vi "Get Module Execution Status.vi"(8 "error in":errorcluster) -> (0 "error out":errorcluster)   [LabVIEW 2025, in "Number Pad.lvlib"]
doc: "Fire the Get Module Execution Status request.\n_____\nBased on DQMH Dev Tools: Project Template 7.1.0.1503."
uses:
  Number Pad.lvlib
  Get Module Execution Status Argument--cluster.ctl
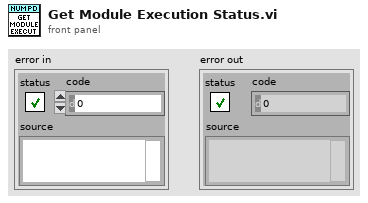
[diagram p1: front panel]
types:
  T1 = typedef "Number Pad.lvlib/Get Module Execution Status Argument--cluster.ctl" = cluster{"Running?":bool}
  T2 = typedef "Number Pad.lvlib/Request Events--cluster.ctl" = cluster{"Stop Module":refnum<user-event>, "Show Panel":refnum<user-event>, "Hide Panel":refnum<user-event>, "Get Module Execution Status":refnum<user-event>, "Show Diagram":refnum<user-event>}
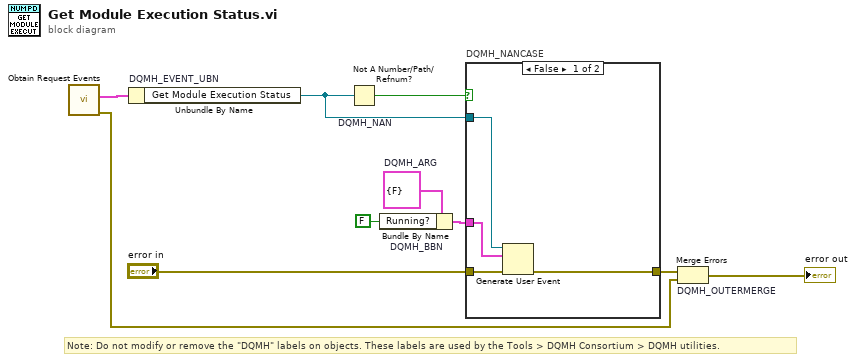
[diagram p0: block diagram]
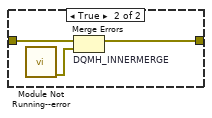
[diagram p2: hidden frame]
diagram:
  w4 = T1 {"Running?"=FALSE}  # DQMH_ARG
  # "Note: Do not modify or remove the \"DQMH\" labels on objects. These labels are used by the Tools > DQMH Consortium > DQMH utilities."
  n1 = call "Obtain Request Events.vi"() -> ("error out"=w2:errorcluster, "Number Pad Request Events"=w1:T2)  [unwired: 10 in]
  n2 = Unbundle By Name "DQMH_EVENT_UBN"(w1) -> ("Get Module Execution Status"=w5:refnum<user-event>)
  n3 = Not A Number/Path/Refnum? "DQMH_NAN"(number/path/refnum=w5) -> (NaN/Path/Refnum?=w6:bool)
  n4 = Bundle By Name "DQMH_BBN"(cluster=w4, "Running?"=FALSE) -> (w7:T1)
  n5 = case "DQMH_NANCASE" shown="False" w6 {
    tunnel: "error in" -> [w14 w17]
    tunnel: [w13 w16] -> w8
    tunnel: w5 -> [w12 _]
    tunnel: w7 -> [w11 _]
    frame False {
      n6 = Generate User Event(user event=w12, event data cluster=w11, error in=w14) -> (error out=w13:errorcluster)  [unwired: 1 in, 1 out]
    }
    frame True {
      n7 = call "Module Not Running--error.vi"() -> ("error out"=w15:errorcluster)  [unwired: 11 in]
      n8 = Merge Errors "DQMH_INNERMERGE"(w17, w15) -> (w16:errorcluster)
    }
  }
  n9 = Merge Errors "DQMH_OUTERMERGE"(w8, w2) -> (→"error out":errorcluster)
